vi "channel_request_pty.vi"() -> ()   [LabVIEW 2017]
doc: "Illustrates how to configure the pseudo-terminal (PTY)."
uses:
  libssh2/libssh2_session_handshake_tcp.vi
  libssh2/libssh2_init_default.vi
  libssh2/libssh2_session_init_ex.vi
  <vilib>/Utility/tcp.llb/TCP Get Raw Net Object.vi
  libssh2/libssh2_session_handshake_socket.vi
  libssh2/libssh2_userauth_password_ex.vi
  libssh2/libssh2_channel_open_ex.vi
  libssh2/libssh2_channel_request_pty_ex.vi
  libssh2/libssh2_channel_process_startup.vi
  libssh2/libssh2_channel_read_ex.vi
  libssh2/libssh2.lvlib
panel:
  in  "term":string(combo)="vt220"
  out "standard output":string
  in  "command":string="tput setaf 1; echo \"test\""
  in  "password":string
  in  "username":string
  out "error out":errorcluster
  in  "hostname":string="localhost"
  # "This is the terminal used.\nFor example, \"xterm\" or \"vt220\".\nNote how the output changes depending on the PTY when formatted text is involved."
  # "This command will produce the text \"test\" in red color."
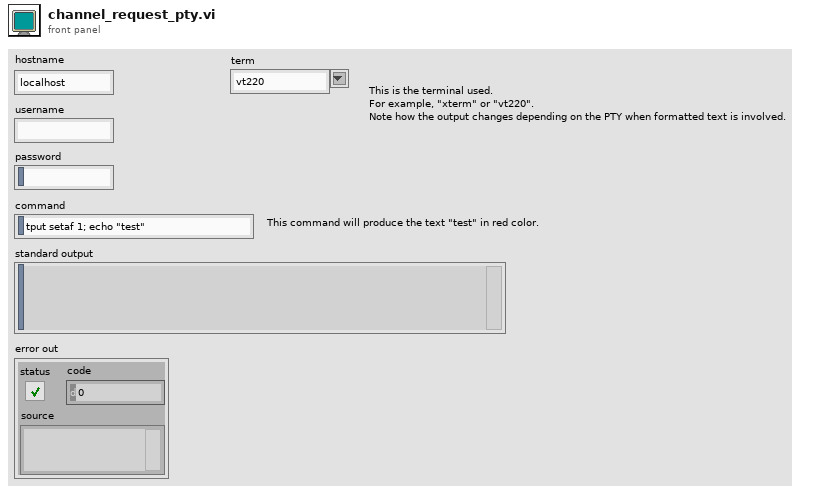
[diagram p1: front panel]
types:
  T1 = typedef "libssh2.lvlib/Session Refnum.ctl" = refnum<k1>
  T2 = typedef "libssh2.lvlib/Channel Refnum.ctl" = refnum<k1>
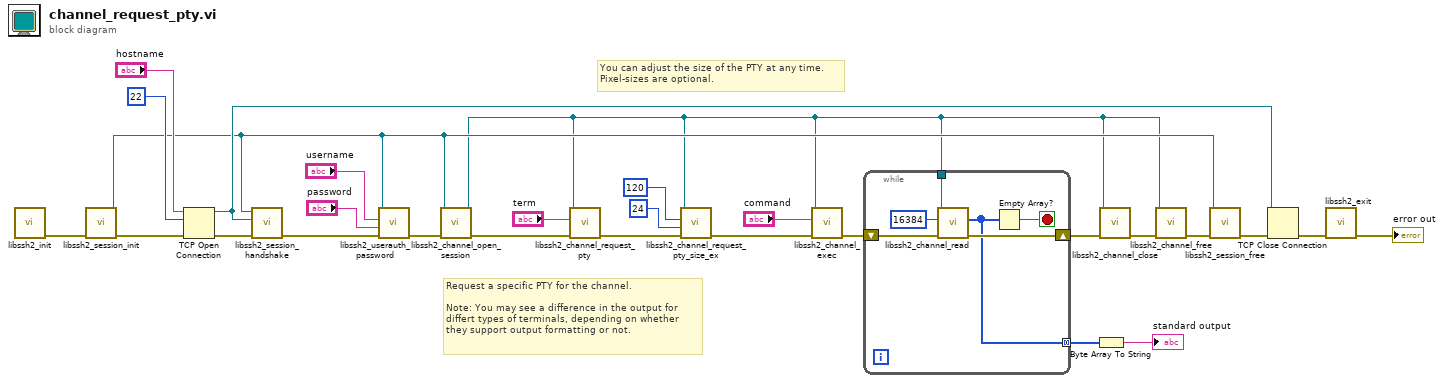
[diagram p0: block diagram]
diagram:
  # "You can adjust the size of the PTY at any time.\nPixel-sizes are optional."
  # "Request a specific PTY for the channel.\n\nNote: You may see a difference in the output for\ndiffert types of terminals, depending on whether\nthey support output formatting or not."
  n1 = call-poly "libssh2_init.vi"() -> ("error out"=w28:errorcluster)  [unwired: 11 in]
  n2 = call "libssh2_session_init.vi"("error in (no error)"=w28) -> ("error out"=w27:errorcluster, "session"=w9:T1)  [unwired: 9 in]
  n3 = TCP Open Connection(address="hostname", remote port or service name=u16 22, error in (no error)=w27) -> (connection ID=w11:refnum<k5>, error out=w12:errorcluster)  [unwired: 2 in]
  n4 = call-poly "libssh2_session_handshake.vi"("error in (no error)"=w12, "tcp connection"=w11, "session"=w9) -> ("error out"=w10:errorcluster)  [unwired: 8 in]
  n5 = call "libssh2_userauth_password.vi"("error in (no error)"=w10, "password"="password", "username"="username", "session"=w9) -> ("error out"=w22:errorcluster)  [unwired: 7 in]
  n6 = call "libssh2_channel_open_session.vi"("error in (no error)"=w22, "session"=w9) -> ("error out"=w19:errorcluster, "channel"=w3:T2)  [unwired: 8 in]
  n7 = call "libssh2_channel_request_pty.vi"("error in (no error)"=w19, "term"="term", "channel"=w3) -> ("error out"=w6:errorcluster)  [unwired: 8 in]
  n8 = call "libssh2_channel_request_pty_size_ex.vi"("error in (no error)"=w6, "height"=24, "width"=120, "channel"=w3) -> ("error out"=w4:errorcluster)  [unwired: 7 in]
  n9 = call "libssh2_channel_exec.vi"("error in (no error)"=w4, "command"="command", "channel"=w3) -> ("error out"=w18:errorcluster)  [unwired: 8 in]
  n10 = while {
    tunnel: w3 -> [w31]
    tunnel: [w29] -> w15 mode=concatenating
    shift-right: [w33] -> w5
    shift-left: w18 -> [w34]
    stop <- w30 stop-if-true
    n11 = call "libssh2_channel_read.vi"("error in (no error)"=w34, "buffer length"=16384 ("buflen"), "channel"=w31) -> ("error out"=w33:errorcluster, "buffer"=w29:u8[])  [unwired: 7 in]
    n12 = Empty Array?(array=w29) -> (empty?=w30:bool)
  }
  n13 = Byte Array To String(unsigned byte array=w15) -> (string=→"standard output":string)
  n14 = call "libssh2_channel_close.vi"("error in (no error)"=w5, "channel"=w3) -> ("error out"=w7:errorcluster)  [unwired: 9 in]
  n15 = call "libssh2_channel_free.vi"("error in (no error)"=w7, "channel"=w3) -> ("error out"=w16:errorcluster)  [unwired: 9 in]
  n16 = call "libssh2_session_free.vi"("error in (no error)"=w16, "session"=w9) -> ("error out"=w26:errorcluster)  [unwired: 9 in]
  n17 = TCP Close Connection(connection ID=w11, error in (no error)=w26) -> (error out=w13:errorcluster)  [unwired: 1 in, 1 out]
  n18 = call "libssh2_exit.vi"("error in (no error)"=w13) -> ("error out"=→"error out":errorcluster)  [unwired: 10 in]
